vi "Close.vi"(8 "error in (no error)":errorcluster, 11 "State Variables in":T1) -> ()   [LabVIEW 2019, in "Instrument Workspace Shared.lvlib"]
uses:
  Instrument Workspace Shared.lvlib
  Types/State Variables.ctl
  <vilib>/NI VeriStand/Execution/Workspace/WorkspaceAPI.ctl
  NationalInstruments.VeriStand.ClientAPI
  NationalInstruments.VeriStand.SystemStorage
  <vilib>/NI VeriStand/Display Template Support/DisplayTemplateSupport.llb/enum_Display Template Handler Minimal To Workspace.ctl
  <vilib>/NI VeriStand/Display Template Support/DisplayTemplateSupport.llb/enum_Display Template Handler Minimal To Widget Msg.ctl
  <vilib>/NI/STM/TCP/TCP Connection Info.ctl
  <vilib>/NI/STM/SubVIs/MetaDataElement.ctl
  Types/CD Saved State.ctl
  <vilib>/NI VeriStand/Execution/Workspace/SystemStateEventRef.ctl
  <vilib>/NI VeriStand/Execution/Workspace/Target State Info.ctl
  <vilib>/NI VeriStand/Execution/Workspace/Target State.ctl
  <vilib>/NI VeriStand/Execution/Workspace/SystemStateRegEventRef.ctl
  <vilib>/NI VeriStand/Execution/Workspace/NI_VS Workspace ExecutionAPI.lvlib
  APIs/Host Automation API/Instrument Host Automation API.lvlib
  <vilib>/NI/STM/NI STM.lvlib
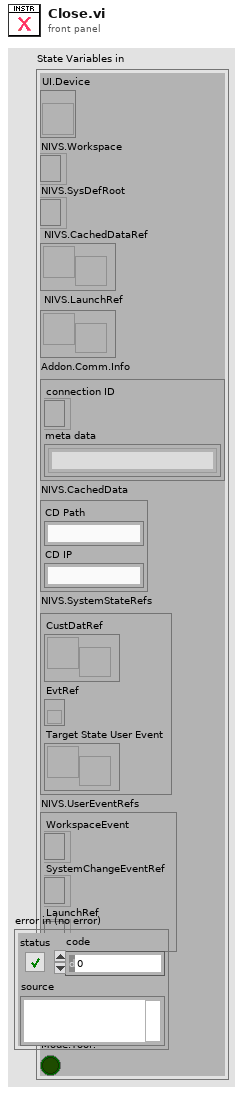
[diagram p1: front panel]
types:
  T1 = typedef "Instrument Workspace Shared.lvlib/State Variables.ctl" = cluster{"UI.Device":refnum<vi>, "NIVS.Workspace":T2, "NIVS.SysDefRoot":refnum<k24>, "NIVS.CachedDataRef":refnum<user-event>, "NIVS.LaunchRef":refnum<user-event>, "Addon.Comm.Info":T3, "NIVS.CachedData":T5, "NIVS.SystemStateRefs":T6, "NIVS.UserEventRefs":cluster{"WorkspaceEvent":refnum<event-registration>, "SystemChangeEventRef":T7, "LaunchRef":refnum<event-registration>}, "NIVS.Workspace Event":refnum<event-registration>, "Addon.Connected?":bool, "Mode.Tool?":bool}
  T2 = typedef "NI_VS Workspace ExecutionAPI.lvlib/WorkspaceAPI.ctl" = refnum<k24>
  T3 = typedef "NI STM.lvlib/TCP Connection Info.ctl" = cluster{"connection ID":refnum<k5>, "meta data":T4[]}
  T4 = typedef "NI STM.lvlib/MetaDataElement.ctl" = string
  T5 = typedef "Instrument Workspace Shared.lvlib/CD Saved State.ctl" = cluster{"CD Path":string, "CD IP":string}
  T6 = typedef "NI_VS Workspace ExecutionAPI.lvlib/SystemStateEventRef.ctl" = cluster{"CustDatRef":refnum<user-event>, "EvtRef":refnum<k27>, "Target State User Event":refnum<user-event>}
  T7 = typedef "NI_VS Workspace ExecutionAPI.lvlib/SystemStateRegEventRef.ctl" = refnum<event-registration>
  T8 = cluster{"WorkspaceEvent":refnum<event-registration>, "SystemChangeEventRef":T7, "LaunchRef":refnum<event-registration>}
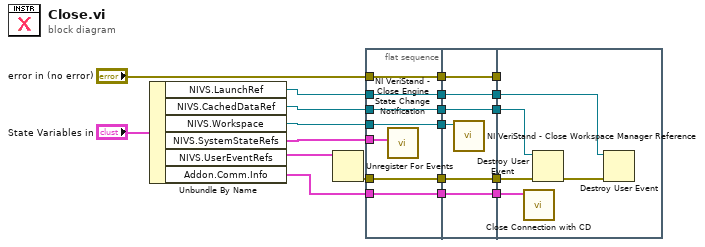
[diagram p0: block diagram]
diagram:
  n1 = Unbundle By Name("State Variables in") -> ("NIVS.LaunchRef"=w8:refnum<user-event>, "NIVS.CachedDataRef"=w7:refnum<user-event>, "NIVS.Workspace"=w6:T2, "NIVS.SystemStateRefs"=w5:T6, "NIVS.UserEventRefs"=w4:T8, "Addon.Comm.Info"=w9:T3)
  n2 = Unregister For Events(event registration refnum=w4) -> (error out=w2:errorcluster)  [unwired: 1 in]
  n3 = flat-sequence {
    tunnel: w9 -> [w23]
    tunnel: w7 -> [w24]
    tunnel: w8 -> [w25]
    tunnel: w2 -> [w26]
    tunnel: "error in (no error)" -> [w27]
    tunnel: [w27] -> w20
    tunnel: [w26] -> w19
    tunnel: [w25] -> w18
    tunnel: [w24] -> w17
    tunnel: [w23] -> w16
    tunnel: w5 -> [w22]
    tunnel: w6 -> [w21]
    tunnel: [w21] -> w15
    tunnel: w20 -> [w33]
    tunnel: [w33] -> w14
    tunnel: w19 -> [w32]
    tunnel: [w32] -> w13
    tunnel: w18 -> [w31]
    tunnel: [w31] -> w12
    tunnel: w17 -> [w30]
    tunnel: [w30] -> w11
    tunnel: w16 -> [w29]
    tunnel: [w29] -> w10
    tunnel: w15 -> [w28]
    tunnel: w14 -> [_]
    tunnel: w13 -> [w35]
    tunnel: w12 -> [w38]
    tunnel: w11 -> [w37]
    tunnel: w10 -> [w36]
    frame #0 {
      n4 = call <vilib>:"NI VeriStand - Close Engine State Change Notification.vi"("SystemStateRefs"=w22) -> ()  [unwired: 10 in, 1 out]
    }
    frame #1 {
      n5 = call <vilib>:"NI VeriStand - Close Workspace Manager Reference.vi"("WorkspaceManager"=w28) -> ()  [unwired: 10 in, 1 out]
    }
    frame #2 {
      n6 = call "Close Connection with CD.vi"("Comm.Info"=w36) -> ()  [unwired: 10 in, 1 out]
      n7 = Destroy User Event(user event=w37, error in=w35) -> (error out=w34:errorcluster)
      n8 = Destroy User Event(user event=w38, error in=w34) -> ()  [unwired: 1 out]
    }
  }
